vi "IDSinit.vi"(7 "error in (no error)":errorcluster, 10 "Camera ID":i32) -> (0 "error out":errorcluster, 1 "Cam Info":T1, 2 "Ranges":T3, 3 "reference out":refnum<k24>)   [LabVIEW 2014]
uses:
  <vilib>/Utility/miscctls.llb/LVMinMaxIncTypeDef.ctl
  C:/Program Files (x86)/National Instruments/LabVIEW 2014/instr.lib/IDS/ueye.NET/uEyeDotNet.dll
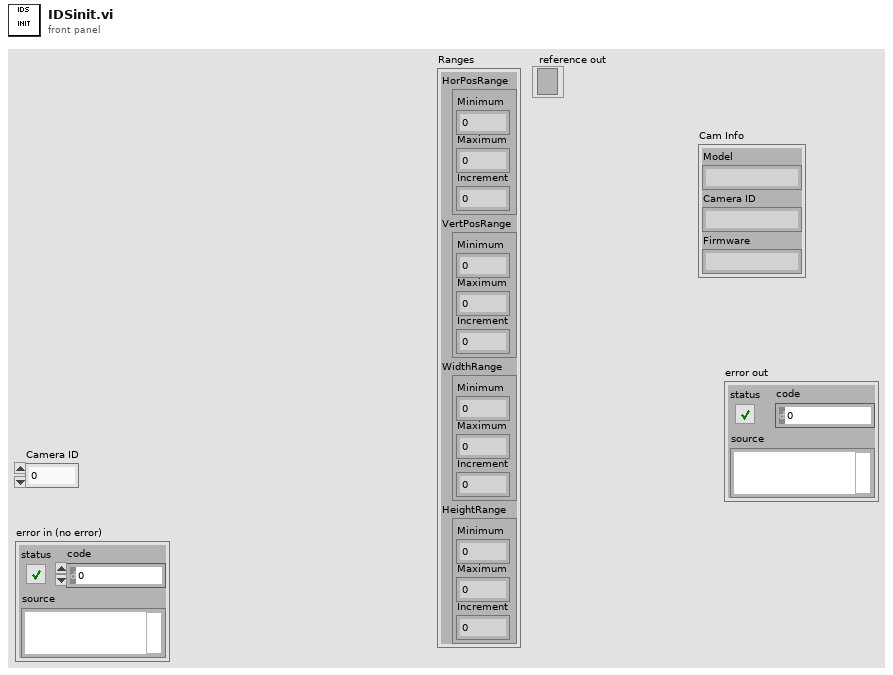
[diagram p1: front panel]
types:
  T1 = cluster{"Model":string, "Camera ID":string, "Firmware":string}
  T2 = typedef "LVMinMaxIncTypeDef.ctl" = cluster{"Minimum":dbl, "Maximum":dbl, "Increment":dbl}
  T3 = cluster{"HorPosRange":T2, "VertPosRange":T2, "WidthRange":T2, "HeightRange":T2}
  T4 = cluster{"Data Entry Limits":T2, "Data Entry Limits":T2, "Data Entry Limits":T2, "Data Entry Limits":T2}
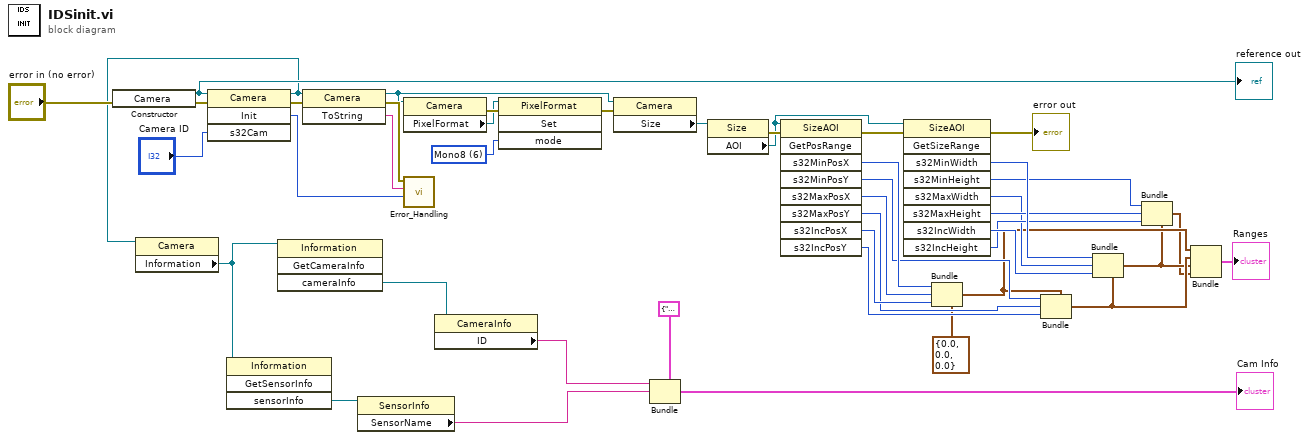
[diagram p0: block diagram]
diagram:
  w10 = 6 items=["BGRA8Packed"=0, "BGR8Packed"=1, "BGR565Packed"=2, "BGR5Packed"=3, "Mono8"=6, "SensorRaw8"=11, "UYVYPacked"=12, "UYVYMonoPacked"=13, "UYVYBayerPacked"=14, "CBYCRYPacked"=23, "BGRY8Packed"=24, "BGR10Packed"=25, "Mono12"=26, "SensorRaw12"=27, "Mono16"=28, "SensorRaw16"=29, "BGR12Unpacked"=30, "BGRA12Unpacked"=31, "Jpeg"=32, "BGR10Unpacked"=35, "RGBA8Packed"=128, "RGB8Packed"=129, "RGBY8Packed"=152, "RGB10Packed"=153, "RGB12Unpacked"=158, "RGBA12Unpacked"=159, "RGB10Unpacked"=163, "RGB8Planar"=8321, "PreferPackedSourceFormat"=16384] ("mode")
  n1 = constructor class="Camera"(error in="error in (no error)") -> (reference out=w9:refnum<k24>, error out=w43:errorcluster)  [unwired: 2 in, 1 out]
  "reference out" <- w9
  n2 = invoke class="Camera" method="Init"(reference=w9, error in=w43, "s32Cam"="Camera ID") -> (reference out=w4:refnum<k24>, error out=w41:errorcluster, "Init"=w39:i32)  [unwired: 1 in, 1 out]
  n3 = property class="Camera"(reference=w4) -> ("Information"=w3:refnum<k24>)  [unwired: 1 in, 2 out]
  n4 = invoke class="Information" method="GetSensorInfo"(reference=w3) -> ("sensorInfo"=w2:refnum<k24>)  [unwired: 3 in, 3 out]
  n5 = invoke class="Information" method="GetCameraInfo"(reference=w3) -> ("cameraInfo"=w8:refnum<k24>)  [unwired: 3 in, 3 out]
  n6 = invoke class="Camera" method="ToString"(reference=w4, error in=w41) -> (reference out=w13:refnum<k24>, error out=w38:errorcluster, "ToString"=w40:string)  [unwired: 1 in]
  n7 = property class="SensorInfo"(reference=w2) -> ("SensorName"=w1:string)  [unwired: 1 in, 2 out]
  n8 = property class="Camera"(reference=w13) -> (error out=w14:errorcluster, "PixelFormat"=w12:refnum<k24>)  [unwired: 1 in, 1 out]
  n9 = call <instrlib>:"Error_Handling.vi"("Error Code"=w39, "Error String"=w40, "Error In"=w38) -> ()  [unwired: 8 in, 1 out]
  n10 = property class="CameraInfo"(reference=w8) -> ("ID"=w6:string)  [unwired: 1 in, 2 out]
  n11 = invoke class="PixelFormat" method="Set"(reference=w12, error in=w14, "mode"=w10) -> (error out=w11:errorcluster)  [unwired: 1 in, 3 out]
  n12 = property class="Camera"(reference=w13, error in=w11) -> ("Size"=w21:refnum<k24>)  [unwired: 2 out]
  n13 = Bundle(cluster=T1 {"Model"="", "Camera ID"="", "Firmware"=""} ("Camera Details"), "Model"=w6, "Camera ID"=w1) -> (→"Cam Info":T1)  [unwired: 1 in]
  n14 = property class="Size"(reference=w21) -> (error out=w30:errorcluster, "AOI"=w28:refnum<k24>)  [unwired: 1 in, 1 out]
  n15 = invoke class="SizeAOI" method="GetPosRange"(reference=w28, error in=w30) -> (error out=w29:errorcluster, "s32MinPosX"=w37:i32, "s32MinPosY"=w34:i32, "s32MaxPosX"=w36:i32, "s32MaxPosY"=w33:i32, "s32IncPosX"=w35:i32, "s32IncPosY"=w32:i32)  [unwired: 7 in, 2 out]
  n16 = invoke class="SizeAOI" method="GetSizeRange"(reference=w28, error in=w29) -> (error out=→"error out":errorcluster, "s32MinWidth"=w25:i32, "s32MinHeight"=w22:i32, "s32MaxWidth"=w20:i32, "s32MaxHeight"=w24:i32, "s32IncWidth"=w26:i32, "s32IncHeight"=w23:i32)  [unwired: 7 in, 2 out]
  n17 = Bundle(cluster=T2 {"Minimum"=0.0, "Maximum"=0.0, "Increment"=0.0} ("Data Entry Limits"), "Minimum"=w37, "Maximum"=w36, "Increment"=w35) -> (w19:T2)
  n18 = Bundle(cluster=w19, "Minimum"=w34, "Maximum"=w33, "Increment"=w32) -> (w18:T2)
  n19 = Bundle(cluster=w18, "Minimum"=w25, "Maximum"=w20, "Increment"=w26) -> (w17:T2)
  n20 = Bundle(cluster=w17, "Minimum"=w22, "Maximum"=w24, "Increment"=w23) -> (w16:T2)
  n21 = Bundle("Data Entry Limits"=w19, "Data Entry Limits"=w18, "Data Entry Limits"=w17, "Data Entry Limits"=w16) -> (→"Ranges":T4)  [unwired: 1 in]
